vi "Get Packet type.vi"(8 "error in (no error)":errorcluster, 11 "niDTS BT Dut in":refnum<class "niDTS BT Dut.lvclass">) -> (0 "error out":errorcluster, 2 "Packet type":T1(ring)=enum."DH1", 3 "niDTS BT Dut out":refnum<class "niDTS BT Dut.lvclass">)   [LabVIEW 2015, in "niDTS BT.lvlib" / "niDTS BT Dut.lvclass"]
uses:
  niDTS BT Dut.lvclass
  niDTS BT Dut.lvclass/niDTS BT Dut.ctl
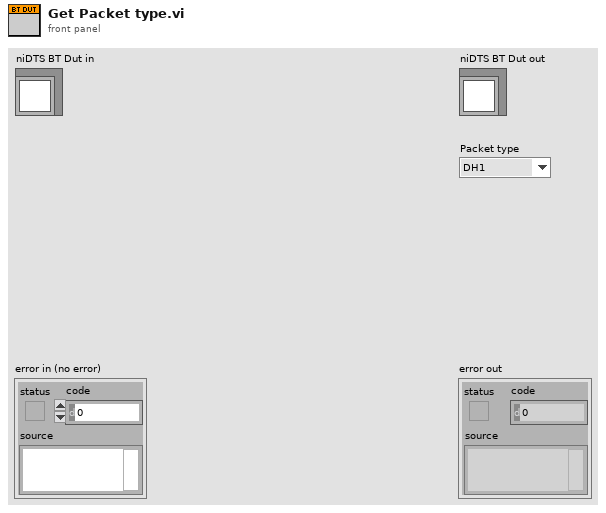
[diagram p1: front panel]
types:
  T1 = enum16{"NULL", "POLL", "FHS", "DM1", "DH1", "HV1", "HV2", "HV3", "EV3", "DV", "AUX1", "DM3", "DH3", "EV4", "EV5", "DM5", "DH5", "LE-TP"}
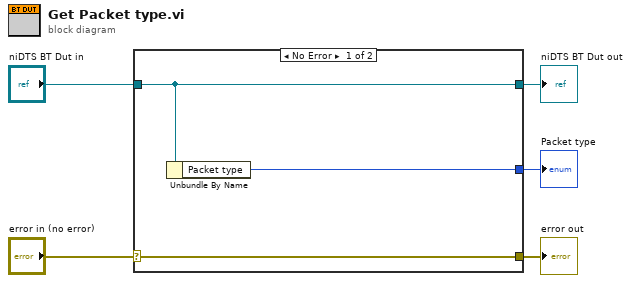
[diagram p0: block diagram]
diagram:
  n1 = case shown="No Error" "error in (no error)" {
    selector: "error in (no error)" -> [w8 w9]
    tunnel: [w8 w9] -> w4
    tunnel: [w7 w10] -> w2
    tunnel: "niDTS BT Dut in" -> [w7 w10]
    tunnel: [w6 _] -> w1
    frame No Error {
      n2 = Unbundle By Name(w7) -> ("Packet type"=w6:T1)
    }
    frame Error {
    }
  }
  "error out" <- w4
  "niDTS BT Dut out" <- w2
  "Packet type" <- w1
